vi "SweepDataEntry.vi"(0 "Enter Stop":bool caption="Stop", 1 "Start ini":dbl=200.0, 2 "Enter Start":bool caption="Start", 3 "Keypad In":dbl, 5 "Stop ini":dbl=4000.0, 9 "Enter ST":bool caption="Stime", 11 "Step ini":dbl=5.0, 12 "Enter SZ":bool caption="Ssize", 13 "SZ ini":dbl=50.0) -> (4 "START FREQUENCY MHz":dbl=200.0 format="%_7g", 6 "STOP FREQUENCY MHz":dbl=4000.0 format="%_7g", 8 "reset":bool, 10 "Step Time mS":dbl=5.0, 15 "Step Size MHz":dbl=50.0 format="%#_7f")   [LabVIEW 2013]
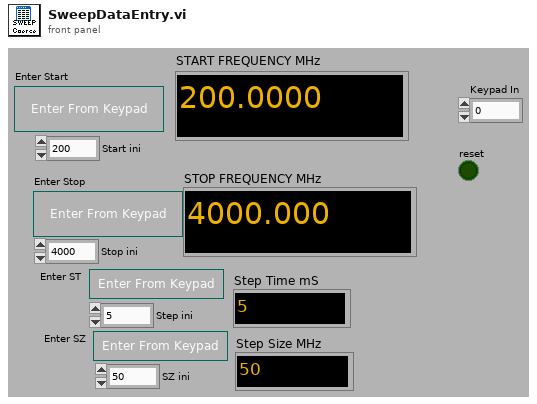
[diagram p1: front panel]
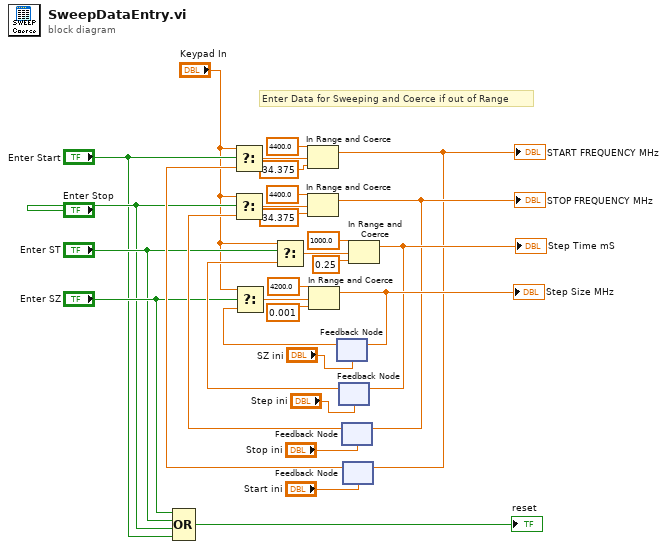
[diagram p0: block diagram]
diagram:
  # "Enter Data for Sweeping and Coerce if out of Range"
  n1 = Compound Arithmetic op=OR("Enter SZ", "Enter ST", "Enter Stop", "Enter Start") -> (→"reset":bool)
  n2 = feedback #1("SZ ini") -> (w20:dbl)
  n3 = Select(t="Keypad In", s="Enter SZ", f=w20) -> (s? t:f=w23:dbl)
  n4 = In Range and Coerce(upper limit=4200.0, x=w23, lower limit=0.001) -> (coerced(x)=w21:dbl)  [unwired: 1 out]
  "Step Size MHz" <- w21
  n5 = feedback-in #1(w21) -> ()
  n6 = feedback #2("Step ini") -> (w17:dbl)
  n7 = Select(t="Keypad In", s="Enter ST", f=w17) -> (s? t:f=w26:dbl)
  n8 = feedback #3("Stop ini") -> (w14:dbl)
  n9 = Select(t="Keypad In", s="Enter Stop", f=w14) -> (s? t:f=w28:dbl)
  n10 = In Range and Coerce(upper limit=4400.0, x=w28, lower limit=34.375) -> (coerced(x)=w15:dbl)  [unwired: 1 out]
  "STOP FREQUENCY MHz" <- w15
  n11 = feedback-in #3(w15) -> ()
  n12 = feedback #4("Start ini") -> (w9:dbl)
  n13 = Select(t="Keypad In", s="Enter Start", f=w9) -> (s? t:f=w11:dbl)
  n14 = In Range and Coerce(upper limit=4400.0, x=w11, lower limit=34.375) -> (coerced(x)=w10:dbl)  [unwired: 1 out]
  "START FREQUENCY MHz" <- w10
  n15 = feedback-in #4(w10) -> ()
  n16 = In Range and Coerce(upper limit=1000.0, x=w26, lower limit=0.25) -> (coerced(x)=w18:dbl)  [unwired: 1 out]
  "Step Time mS" <- w18
  n17 = feedback-in #2(w18) -> ()
